vi "StateBallHandling.vi"(7 "Master State":enum16{"Normal", "Climb"}(ring), 13 "Shooter Firing":bool) -> ()   [LabVIEW 2020]
doc: "This VI makes all decisions related to the ball handling subsystems including the intake, indexer, and tower."
uses:
  sensordata.vi
  driverdata.vi
  drivercommands.vi
  autonomousinfo.vi
  robotoutputs.vi
panel:
  in  "Tower Power When Shooting":dbl=0.3
  in  "Indexer Threshold (ms)":u32
  in  "Intake Delay (ms)":u32=1000
  in  "Tower Power":dbl=0.2
  in  "Indexer Power":dbl=0.4
  in  "Intake Power":dbl=0.4
  out "Ball Handling State":u32
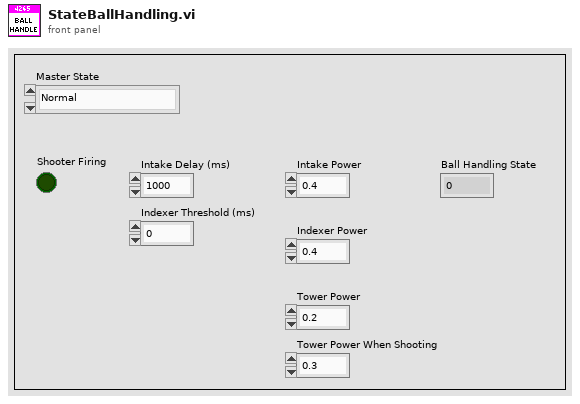
[diagram p1: front panel]
types:
  T1 = enum16{"Robot-Oriented", "Field-Oriented", "Intake"}
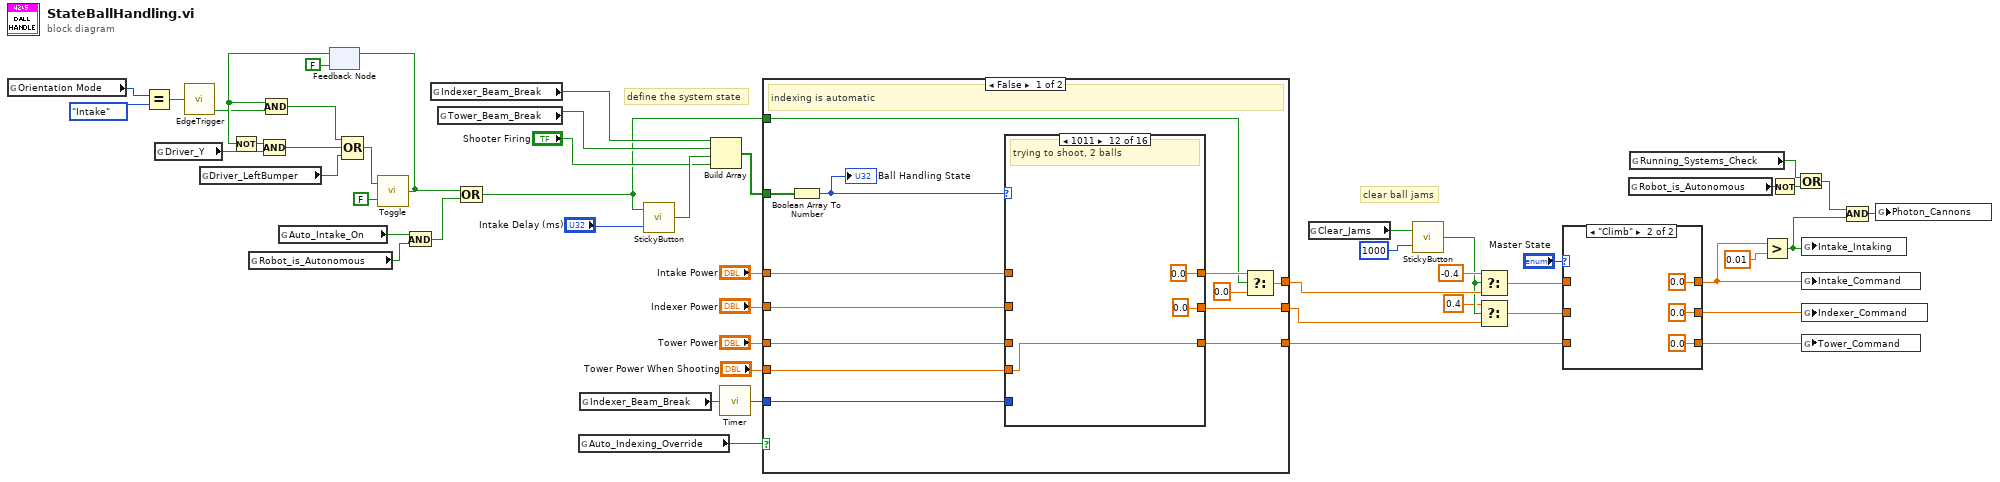
[diagram p0: block diagram]
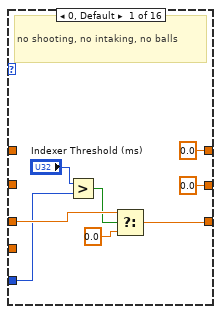
[diagram p3: hidden frame]
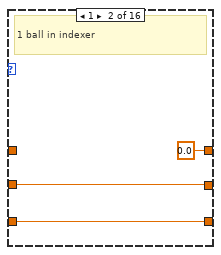
[diagram p4: hidden frame]
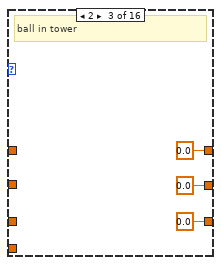
[diagram p5: hidden frame]
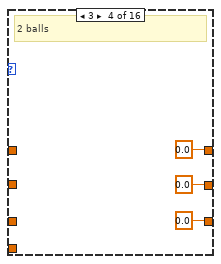
[diagram p6: hidden frame]
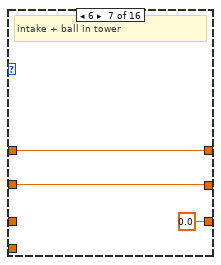
[diagram p9: hidden frame]
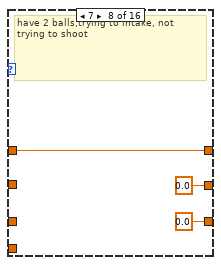
[diagram p10: hidden frame]
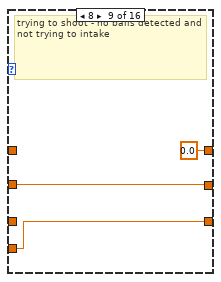
[diagram p11: hidden frame]
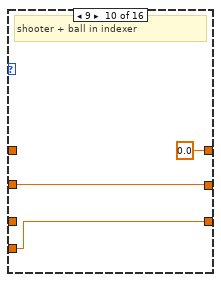
[diagram p12: hidden frame]
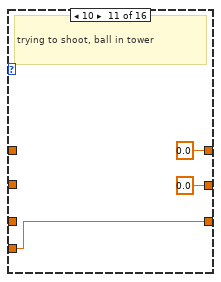
[diagram p13: hidden frame]
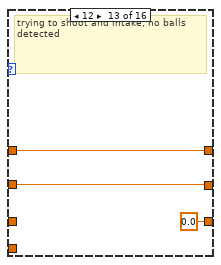
[diagram p14: hidden frame]
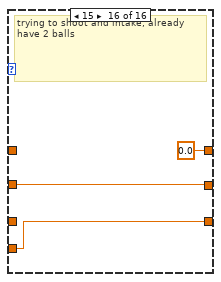
[diagram p17: hidden frame]
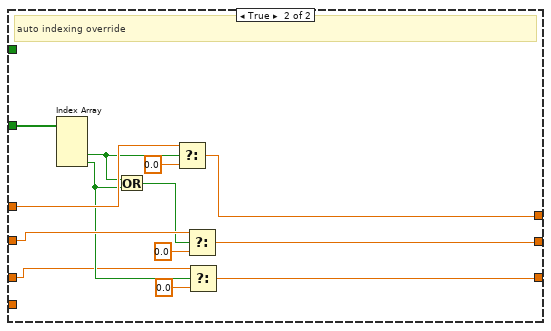
[diagram p18: hidden frame]
diagram:
  # "clear ball jams"
  # "define the system state"
  n1 = global read "robotoutputs.vi" "Orientation Mode"() -> (w9:T1)
  n2 = Equal?(x=w9, y=T1."Intake" ("Orientation Mode")) -> (x = y?=w2:bool)
  n3 = global read "drivercommands.vi" "Driver_Y"() -> (w13:bool)
  n4 = call "EdgeTrigger.vi"("Input Signal"=w2) -> ("Falling Edge Trigger"=w1:bool)  [unwired: 2 out]
  n5 = global read "drivercommands.vi" "Driver_LeftBumper"() -> (w12:bool)
  n6 = global read "driverdata.vi" "Robot_is_Autonomous"() -> (w23:bool)
  n7 = global read "autonomousinfo.vi" "Auto_Intake_On"() -> (w24:bool)
  n8 = feedback #1(FALSE ("New State")) -> (w4:bool)
  n9 = Not(x=w4) -> (.not. x?=w6:bool)
  n10 = Compound Arithmetic op=AND(w6, w13) -> (w5:bool)
  n11 = Compound Arithmetic op=AND(w4, w1) -> (w3:bool)
  n12 = Compound Arithmetic op=OR(w3, w5, w12) -> (w10:bool)
  n13 = call "Toggle.vi"("Initial State"=FALSE, "Trigger"=w10) -> ("New State"=w7:bool)
  n14 = feedback-in #1(w7) -> ()
  n15 = And(x=w24, y=w23) -> (x .and. y?=w22:bool)
  n16 = global read "sensordata.vi" "Indexer_Beam_Break"() -> (w47:bool)
  n17 = global read "sensordata.vi" "Tower_Beam_Break"() -> (w48:bool)
  n18 = Compound Arithmetic op=OR(w7, w22) -> (w15:bool)
  n19 = global read "driverdata.vi" "Auto_Indexing_Override"() -> (w41:bool)
  n20 = global read "sensordata.vi" "Indexer_Beam_Break"() -> (w43:bool)
  n21 = call "StickyButton.vi"("Time threshold (ms)"="Intake Delay (ms)", "Button Input"=w15) -> ("Sticky Button"=w45:bool)
  n22 = Build Array(w47, w48, w45, "Shooter Firing") -> (w40:bool[])
  n23 = call "Timer.vi"("Reset Timer"=w43) -> ("Time (ms)"=w42:u32)
  n24 = case shown="False" w41 {
    tunnel: "Intake Power" -> [w65 w130]
    tunnel: "Indexer Power" -> [w64 w129]
    tunnel: "Tower Power" -> [w63 w121]
    tunnel: [w62 w125] -> w27
    tunnel: [w61 w119] -> w36
    tunnel: [w58 w126] -> w32
    tunnel: w15 -> [w57 _]
    tunnel: w42 -> [w56 _]
    tunnel: w40 -> [w55 w131]
    tunnel: "Tower Power When Shooting" -> [w53 _]
    frame False {
      # "indexing is automatic"
      n25 = Boolean Array To Number(Boolean array=w55) -> (number=w54:u32)
      "Ball Handling State" <- w54
      n26 = case shown="1011" w54 {
        tunnel: [0.0 0.0 0.0 0.0 w85 w88 w91 w92 0.0 ("Intake Power") 0.0 ("Intake Power") 0.0 ("Intake Power") 0.0 ("Intake Power") w109 w112 w115 0.0 ("Intake Power")] -> w60
        tunnel: [0.0 w76 0.0 0.0 w84 w87 w90 0.0 ("Indexer Power") w97 w100 0.0 ("Indexer Power") 0.0 ("Indexer Power") w108 w111 w114 w118] -> w62
        tunnel: [w69 w75 0.0 0.0 w83 w86 0.0 ("Tower Power") 0.0 ("Tower Power") w95 w98 w101 w105 0.0 ("Tower Power") w110 w113 w116] -> w61
        tunnel: w65 -> [_ _ _ _ w85 w88 w91 w92 _ _ _ _ w109 w112 w115 _]
        tunnel: w64 -> [_ w76 _ _ w84 w87 w90 _ w97 w100 _ _ w108 w111 w114 w118]
        tunnel: w63 -> [w71 w75 _ _ w83 w86 _ _ _ _ _ _ _ _ _ _]
        tunnel: w56 -> [w67 _ _ _ _ _ _ _ _ _ _ _ _ _ _ _]
        tunnel: w53 -> [_ _ _ _ _ _ _ _ w95 w98 w101 w105 _ w110 w113 w116]
        frame 0, Default {
          # "no shooting, no intaking, no balls"
          n27 = Greater?(x="Indexer Threshold (ms)", y=w67) -> (0:w68:bool)
          n28 = Select(t=w71, s=w68, f=0.0) -> (s? t:f=w69:dbl)
        }
        frame 1 {
          # "1 ball in indexer"
        }
        frame 2 {
          # "ball in tower"
        }
        frame 3 {
          # "2 balls"
        }
        frame 4 {
          # "intake + no balls"
        }
        frame 5 {
          # "intaking + ball in indexer"
        }
        frame 6 {
          # "intake + ball in tower"
        }
        frame 7 {
          # "have 2 balls,trying to intake, not trying to shoot"
        }
        frame 8 {
          # "trying to shoot - no balls detected and not trying to intake"
        }
        frame 9 {
          # "shooter + ball in indexer"
        }
        frame 10 {
          # "trying to shoot, ball in tower"
        }
        frame 11 {
          # "trying to shoot, 2 balls"
        }
        frame 12 {
          # "trying to shoot and intake, no balls detected"
        }
        frame 13 {
          # "1 ball in indexer, trying to shoot and intake"
        }
        frame 14 {
          # "ball in shooter, trying to shoot and intake"
        }
        frame 15 {
          # "trying to shoot and intake, already have 2 balls"
        }
      }
      n29 = Select(t=w60, s=w57, f=0.0) -> (s? t:f=w58:dbl)
    }
    frame True {
      # "auto indexing override"
      n30 = Index Array(array=w131) -> (element #3=w124:bool, element #4=w122:bool)  [unwired: 4 in, 2 out]
      n31 = Or(x=w124, y=w122) -> (x .or. y?=w123:bool)
      n32 = Select(t=w130, s=w124, f=0.0) -> (s? t:f=w126:dbl)
      n33 = Select(t=w129, s=w123, f=0.0) -> (s? t:f=w125:dbl)
      n34 = Select(t=w121, s=w122, f=0.0) -> (s? t:f=w119:dbl)
    }
  }
  n35 = global read "drivercommands.vi" "Clear_Jams"() -> (w34:bool)
  n36 = call "StickyButton.vi"("Time threshold (ms)"=u32 1000, "Button Input"=w34) -> ("Sticky Button"=w28:bool)
  n37 = Select(t=-0.4, s=w28, f=w32) -> (s? t:f=w31:dbl)
  n38 = Select(t=0.4, s=w28, f=w27) -> (s? t:f=w29:dbl)
  n39 = case shown="\"Climb\"" "Master State" {
    tunnel: w31 -> [w134 _]
    tunnel: [w134 0.0 ("f")] -> w38
    tunnel: [w133 0.0 ("f")] -> w37
    tunnel: w29 -> [w133 _]
    tunnel: w36 -> [w132 _]
    tunnel: [w132 0.0 ("f")] -> w35
    frame "Normal", Default {
    }
    frame "Climb" {
    }
  }
  n40 = global read "driverdata.vi" "Robot_is_Autonomous"() -> (w19:bool)
  n41 = global read "driverdata.vi" "Running_Systems_Check"() -> (w17:bool)
  n42 = Greater?(x=w38, y=0.01) -> (0:w20:bool)
  n43 = Not(x=w19) -> (.not. x?=w18:bool)
  n44 = Or(x=w17, y=w18) -> (x .or. y?=w16:bool)
  n45 = global write "robotoutputs.vi" "Intake_Intaking"(w20) -> ()
  n46 = global write "robotoutputs.vi" "Intake_Command"(w38) -> ()
  n47 = global write "robotoutputs.vi" "Indexer_Command"(w37) -> ()
  n48 = global write "robotoutputs.vi" "Tower_Command"(w35) -> ()
  n49 = Compound Arithmetic op=AND(w16, w20) -> (w21:bool)
  n50 = global write "robotoutputs.vi" "Photon_Cannons"(w21) -> ()
